vi "Read Unregister result notifier.vi"(8 "error in (no error)":errorcluster, 11 "Unregister JSON in":refnum<class "Unregister JSON.lvclass">) -> (0 "error out":errorcluster, 2 "Unregister result notifier":refnum<notifier>, 3 "Unregister JSON out":refnum<class "Unregister JSON.lvclass">)   [LabVIEW 2020, in "wamplv.lvlib" / "Unregister JSON.lvclass"]
uses:
  Unregister JSON.lvclass
  Unregister JSON.lvclass/Unregister JSON.ctl
  WAMP Client/API/TypeDefs/Error or abort detail (JSON).ctl
  wamplv.lvlib
  WAMP Client/Private/TypeDef/Success or error (JSON).ctl
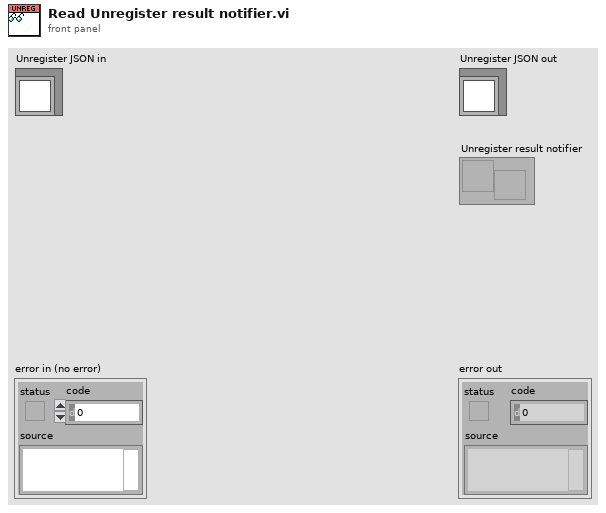
[diagram p1: front panel]
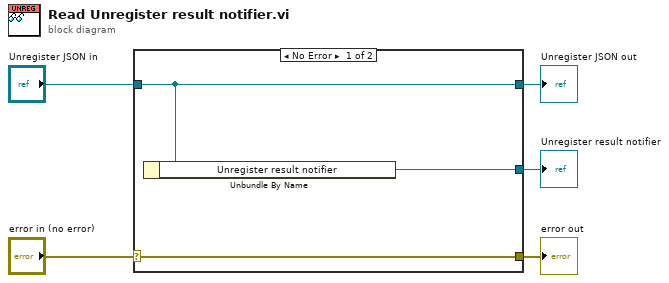
[diagram p0: block diagram]
diagram:
  n1 = case shown="No Error" "error in (no error)" {
    selector: "error in (no error)" -> [w8 w9]
    tunnel: [w8 w9] -> w4
    tunnel: [w7 w10] -> w2
    tunnel: "Unregister JSON in" -> [w7 w10]
    tunnel: [w6 _] -> w1
    frame No Error {
      n2 = Unbundle By Name(w7) -> ("Unregister result notifier"=w6:refnum<notifier>)
    }
    frame Error {
    }
  }
  "error out" <- w4
  "Unregister JSON out" <- w2
  "Unregister result notifier" <- w1
